vi "fireAlarm.vi"() -> ()   [LabVIEW 2018]
panel:
  out "ALARM":bool
  in  "THERMOMETER":dbl(slide) scale=-20.0..100.0
  in  "ON/OFF\nBUTTON":bool
  out "SMOKE ALARM":bool
  out "TEMPERATURE ALARM":bool
  in  "SMOKE  LEVEL SET POINT":dbl(slide) scale=0.0..100.0
  in  "SMOKE LEVEL DETECTOR":dbl(slide) scale=0.0..100.0
  in  "TEMP SET POINT":dbl(slide) scale=-20.0..100.0
  # "FIRE ALARM SYSTEM  (FRONT PANEL)"
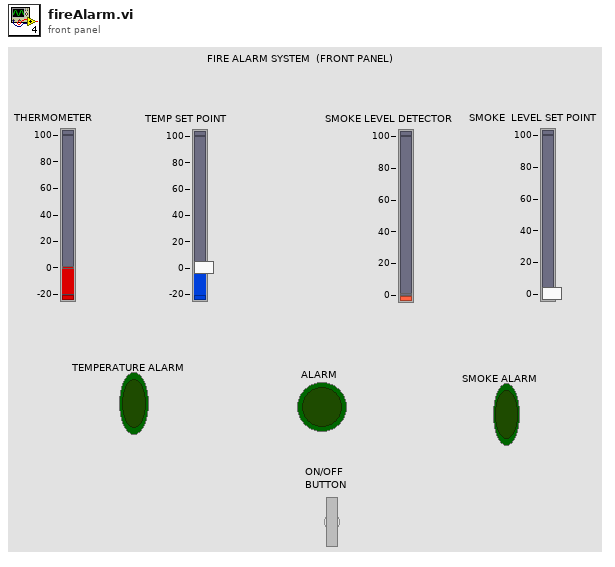
[diagram p1: front panel]
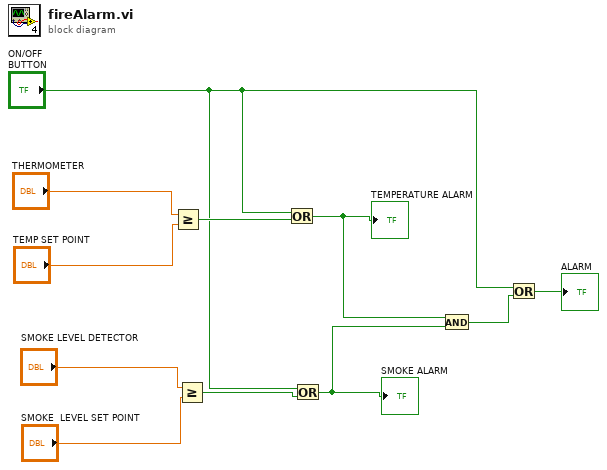
[diagram p0: block diagram]
diagram:
  n1 = Greater Or Equal?(x="THERMOMETER", y="TEMP SET POINT") -> (x >= y?=w9:bool)
  n2 = Greater Or Equal?(x="SMOKE LEVEL DETECTOR", y="SMOKE  LEVEL SET POINT") -> (x >= y?=w6:bool)
  n3 = Or(x="ON/OFF\nBUTTON", y=w9) -> (x .or. y?=w4:bool)
  "TEMPERATURE ALARM" <- w4
  n4 = Or(x="ON/OFF\nBUTTON", y=w6) -> (x .or. y?=w3:bool)
  "SMOKE ALARM" <- w3
  n5 = And(x=w4, y=w3) -> (x .and. y?=w2:bool)
  n6 = Or(x="ON/OFF\nBUTTON", y=w2) -> (x .or. y?=→"ALARM":bool)
